vi "RotatePath.vi"(8 "Angle":sgl, 11 "Path":T2) -> (3 "RotatedPath":T2)   [LabVIEW 2014]
uses:
  TypeDefs/Point2DwSlope.ctl
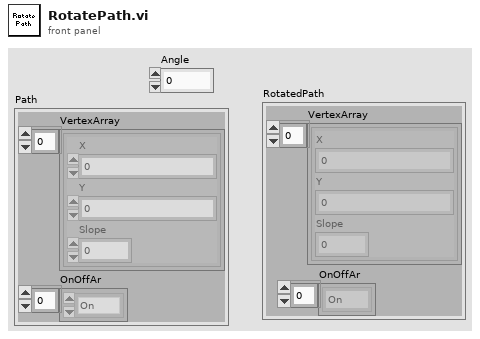
[diagram p1: front panel]
types:
  T1 = typedef "Point2DwSlope.ctl" = cluster{"X":sgl, "Y":sgl, "Slope":dbl}
  T2 = cluster{"VertexArray":T1[], "OnOffAr":enum16{"On", "Off"}[]}
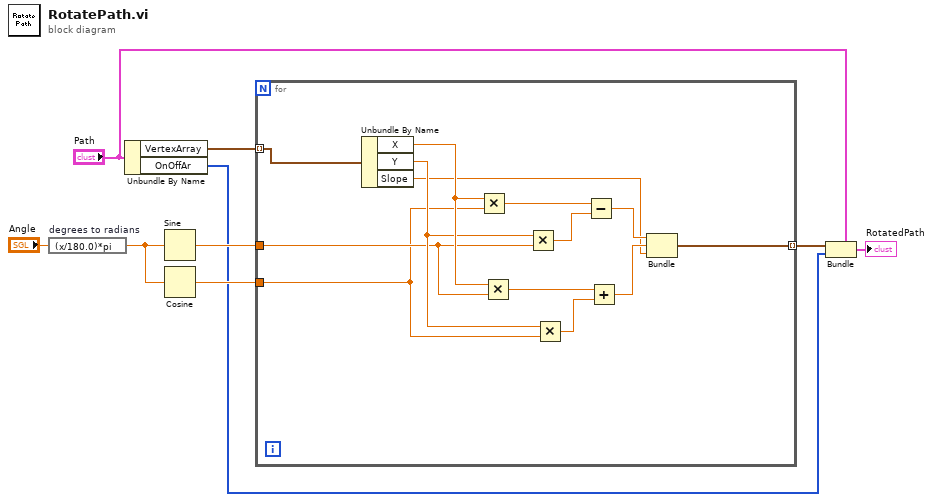
[diagram p0: block diagram]
diagram:
  n1 = expression code="(x/180.0)*pi" "degrees to radians"("Angle") -> (w9:sgl)
  n2 = Unbundle By Name("Path") -> ("VertexArray"=w7:T1[], "OnOffAr"=w3:enum16{"On", "Off"}[])
  n3 = Sine(x=w9) -> (sin(x)=w6:sgl)
  n4 = Cosine(x=w9) -> (cos(x)=w5:sgl)
  n5 = for {
    tunnel: w7 -> [w13] mode=indexing
    tunnel: w6 -> [w12]
    tunnel: w5 -> [w11]
    tunnel: [w10] -> w4 mode=indexing
    n6 = Unbundle By Name(w13) -> ("X"=w20:sgl, "Y"=w18:sgl, "Slope"=w14:dbl)
    n7 = Multiply(x=w20, y=w11) -> (x*y=w22:sgl)
    n8 = Multiply(x=w20, y=w12) -> (x*y=w19:sgl)
    n9 = Multiply(x=w18, y=w12) -> (x*y=w21:sgl)
    n10 = Multiply(x=w18, y=w11) -> (x*y=w17:sgl)
    n11 = Subtract(x=w22, y=w21) -> (x-y=w16:sgl)
    n12 = Add(x=w19, y=w17) -> (x+y=w15:sgl)
    n13 = Bundle(w16, w15, "Slope"=w14) -> (w10:cluster{sgl, sgl, "Slope":dbl})  [unwired: 1 in]
  }
  n14 = Bundle(cluster="Path", "VertexArray"=w4, "OnOffAr"=w3) -> (→"RotatedPath":T2)
